vi "Add Package to SystemLink Feed (By File).vi"(0 "SystemLink repo in":T1, 5 "feed name in":string, 7 "package filepath":path, 9 "timeout (ms) (10000)":u32=10000, 11 "error in (no error)":errorcluster) -> (4 "SystemLink repo out":T1, 6 "feed name out":string, 10 "timed out?":bool, 15 "error out":errorcluster)   [LabVIEW 2017, in "SystemLink_Repo_API.lvlib"]
doc: "Uploads the package to the SystemLink repository, adds the package to the specified feed, and waits for completion.\n\nError Handling:\nOutputs Error 6000 if the upload job fails.\nOutputs Error 6001 if the upload job does not return a status of \"succeeded\" or \"failed\" within the timeout period."
uses:
  SystemLink_Repo_API.lvlib
  <vilib>/httpClient/ClientHandle.ctl
  <vilib>/httpClient/LabVIEWHTTPClient.lvlib
  _support/systemlink repo.ctl
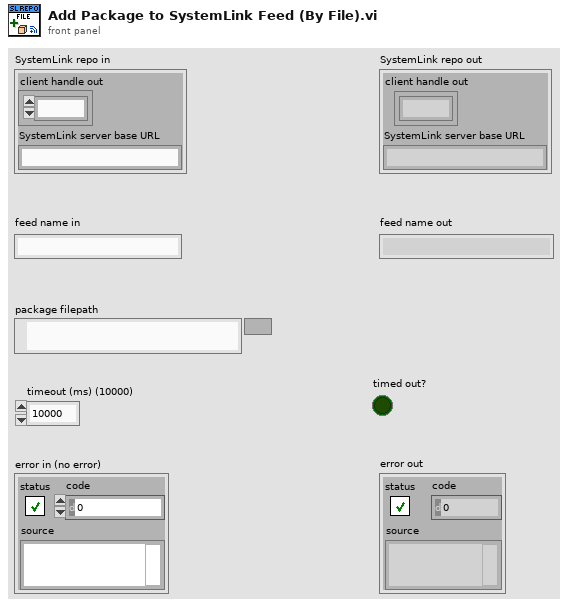
[diagram p1: front panel]
types:
  T1 = typedef "SystemLink_Repo_API.lvlib/systemlink repo.ctl" = cluster{"client handle out":T2, "SystemLink server base URL":string}
  T2 = typedef "LabVIEWHTTPClient.lvlib/ClientHandle.ctl" = refnum<k1>
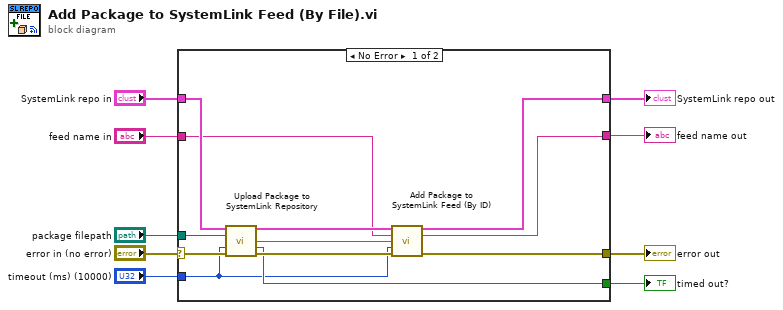
[diagram p0: block diagram]
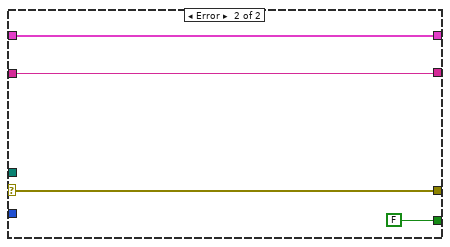
[diagram p2: hidden frame]
diagram:
  n1 = case shown="No Error" "error in (no error)" {
    selector: "error in (no error)" -> [w20 w25]
    tunnel: "SystemLink repo in" -> [w19 w24]
    tunnel: [w12 w25] -> w7
    tunnel: "package filepath" -> [w21 _]
    tunnel: [w16 w23] -> w4
    tunnel: "feed name in" -> [w17 w23]
    tunnel: [w15 w24] -> w3
    tunnel: "timeout (ms) (10000)" -> [w10 _]
    tunnel: [w11 FALSE ("timed out?")] -> w1
    frame No Error {
      n2 = call "Upload Package to SystemLink Repository.vi"("SystemLink repo in"=w19, "package filepath"=w21, "timeout (ms) (10000)"=w10, "error in (no error)"=w20) -> ("SystemLink repo out"=w18:T1, "package ID"=w14:string, "timed out?"=w11:bool, "error out"=w13:errorcluster)  [unwired: 8 in]
      n3 = call "Add Package to SystemLink Feed (By ID).vi"("SystemLink repo in"=w18, "feed name in"=w17, "package ID"=w14, "timeout (ms) (10000)"=w10, "error in (no error)"=w13) -> ("SystemLink repo out"=w15:T1, "feed name out"=w16:string, "error out"=w12:errorcluster)  [unwired: 7 in, 1 out]
    }
    frame Error {
    }
  }
  "error out" <- w7
  "SystemLink repo out" <- w3
  "feed name out" <- w4
  "timed out?" <- w1
